vi "Fetch Measurement (Multiple Point).vi"(8 "error in (no error)":errorcluster, 9 "Data Type (0: Current)":i32(ring) items=["Current", "Status", "Time", "Charge", "Humidity", "Resistance", "Source", "Temperature", "Voltage"], 10 "Channel (1: Channel 1)":i32(ring)=1 items=["Channel 1"=1], 11 "VISA resource name":refnum<visa-resource-name>) -> (0 "error out":errorcluster, 2 "Measurements":dbl[](array[numeric]), 3 "VISA resource name out":refnum<visa-resource-name>)   [LabVIEW 2017, in "Keysight B2980 Series.lvlib"]
doc: "Returns the array data which contains all of the charge measurement data, current measurement data, resistance measurement data, source output setting data, status data, time data, or voltage measurement data.\n\n<B>Note(s):</B>\nUse this VI only with other low-level VIs. The high-level VIs automatically incorporate this functionality. This VI does not check the instrument status."
uses:
  Keysight B2980 Series.lvlib
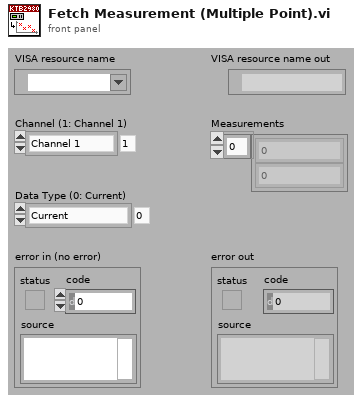
[diagram p1: front panel]
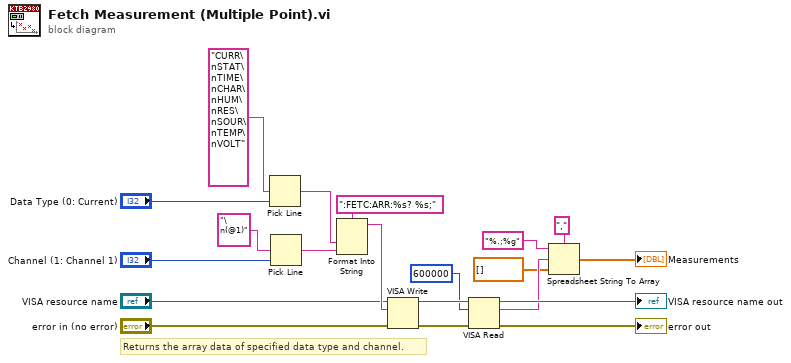
[diagram p0: block diagram]
diagram:
  # "Returns the array data of specified data type and channel."
  n1 = Pick Line(multi-line string="CURR\nSTAT\nTIME\nCHAR\nHUM\nRES\nSOUR\nTEMP\nVOLT", line index="Data Type (0: Current)") -> (output string=w17:string)  [unwired: 1 out]
  n2 = Pick Line(multi-line string="\n(@1)", line index="Channel (1: Channel 1)") -> (output string=w11:string)  [unwired: 1 out]
  n3 = Format Into String(format string=":FETC:ARR:%s? %s;", w17, w11) -> (resulting string=w16:string)  [unwired: 2 in, 1 out]
  n4 = VISA Write(VISA resource name="VISA resource name", write buffer=w16, error in (no error)="error in (no error)") -> (VISA resource name out=w10:refnum<visa-resource-name>, error out=w9:errorcluster)  [unwired: 1 out]
  n5 = VISA Read(VISA resource name=w10, byte count=u32 600000, error in (no error)=w9) -> (VISA resource name out=→"VISA resource name out":refnum<visa-resource-name>, read buffer=w4:string, error out=→"error out":errorcluster)  [unwired: 1 out]
  n6 = Spreadsheet String To Array(delimiter (Tab)=",", format string="%.;%g", spreadsheet string=w4, array type (2D Dbl)=dbl[] []) -> (array=→"Measurements":dbl[])
